vi "Generate_Program_Queue.vi"(2 "error in (no error)":errorcluster, 3 "File Path":path, 4 "Queue in":refnum<queue>) -> (0 "error out":errorcluster, 1 "Queue out":refnum<queue>)   [LabVIEW 2018]
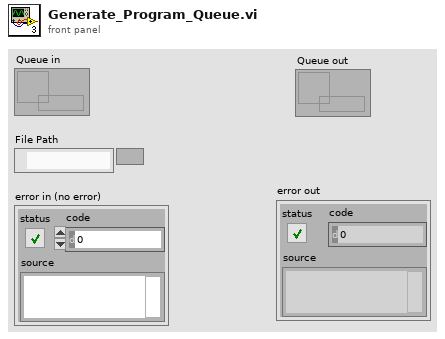
[diagram p1: front panel]
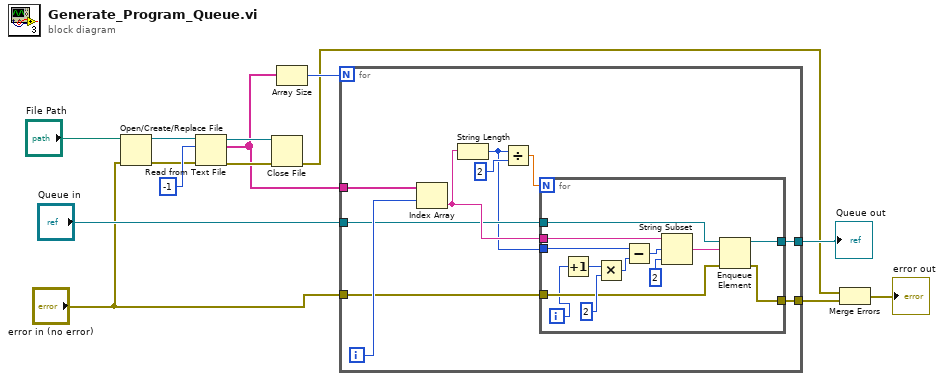
[diagram p0: block diagram]
diagram:
  n1 = Open/Create/Replace File(file path (use dialog)="File Path", error in="error in (no error)") -> (refnum out=w14:refnum<file>, error out=w12:errorcluster)  [unwired: 4 in, 1 out]
  n2 = Read from Text File(file (use dialog)=w14, count=-1, error in=w12) -> (refnum out=w11:refnum<file>, text=w9:string[], error out=w10:errorcluster)  [unwired: 1 in, 1 out]
  n3 = Close File(refnum=w11, error in=w10) -> (error out=w2:errorcluster)  [unwired: 1 out]
  n4 = Array Size(array=w9) -> (size(s)=w8:i32)
  n5 = for {
    N: w8 -> [_]
    tunnel: w9 -> [w24]
    tunnel: "Queue in" -> [w19]
    tunnel: "error in (no error)" -> [w18]
    tunnel: [w17] -> w4
    tunnel: [w16] -> w3
    i -> [w23]
    n6 = Index Array(array=w24, index=w23) -> (element=w20:string)
    n7 = String Length(string=w20) -> (length=w15:i32)
    n8 = Divide(x=w15, y=2) -> (x/y=w21:dbl)
    n9 = for {
      N: w21 -> [_]
      tunnel: w20 -> [w37]
      tunnel: w19 -> [w33]
      tunnel: w18 -> [w32]
      tunnel: [w31] -> w17
      tunnel: [w30] -> w16
      tunnel: w15 -> [w29]
      i -> [w26]
      n10 = Increment(x=w26) -> (x+1=w27:i32)
      n11 = Multiply(x=w27, y=2) -> (x*y=w28:i32)
      n12 = Subtract(x=w29, y=w28) -> (x-y=w25:i32)
      n13 = String Subset(string=w37, offset (0)=w25, length (rest)=2) -> (substring=w34:string)
      n14 = Enqueue Element(queue=w33, element=w34, error in (no error)=w32) -> (queue out=w31:refnum<queue>, error out=w30:errorcluster)  [unwired: 1 in, 1 out]
    }
  }
  "Queue out" <- w4
  n15 = Merge Errors(w2, w3) -> (→"error out":errorcluster)
